vi "LINAKParseStatus.vi"(8 "Error In":errorcluster, 10 "Registers":u16[](array[numeric])) -> (0 "Error Out":errorcluster, 3 "StatusCluster":T1, 4 "GoodToGo":bool)   [LabVIEW 2018]
uses:
  LINAKStatusCluster.ctl
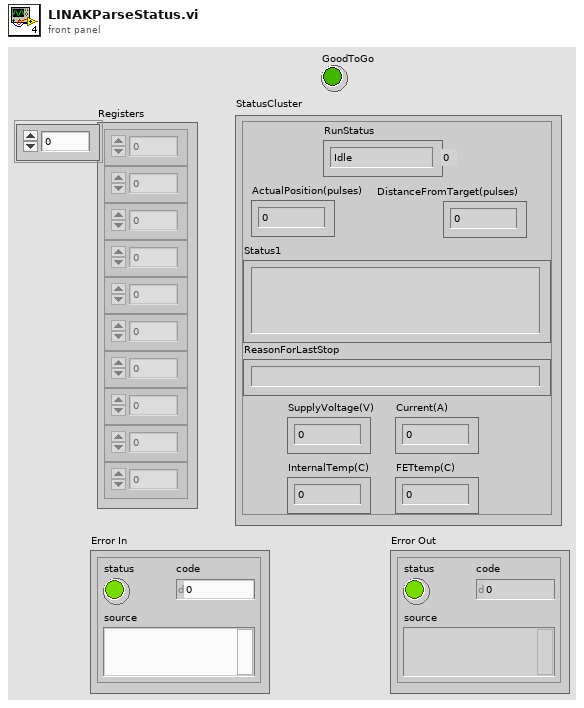
[diagram p1: front panel]
types:
  T1 = typedef "LINAKStatusCluster.ctl" = cluster{"RunStatus":enum16{"Idle", "RunningOut", "RunningIn", "WaitingToRun", "InitOut", "InitIn"}, "ActualPosition(pulses)":u16, "DistanceFromTarget(pulses)":u16, "Status1":string, "ReasonForLastStop":string, "SupplyVoltage(V)":dbl, "Current(A)":dbl, "InternalTemp(C)":i16, "FETtemp(C)":i16}
  T2 = enum16{"Idle", "RunningOut", "RunningIn", "WaitingToRun", "InitOut", "InitIn"}
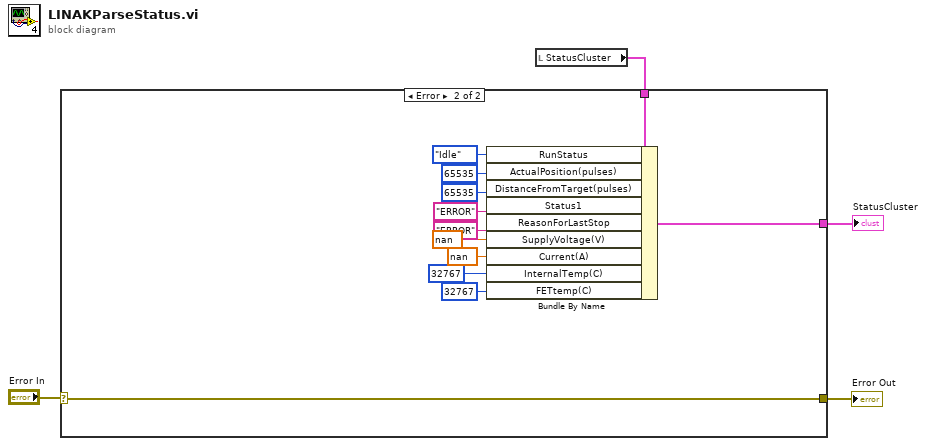
[diagram p0: block diagram]
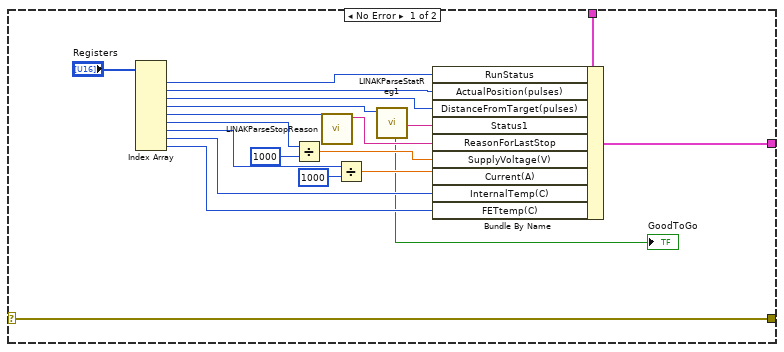
[diagram p2: hidden frame]
diagram:
  n1 = local read "StatusCluster"() -> (w4:T1)
  n2 = case shown="Error" "Error In" {
    selector: "Error In" -> [w5 w25]
    tunnel: w4 -> [w7 w27]
    tunnel: [w6 w26] -> w3
    tunnel: [w5 w25] -> w1
    frame No Error {
      n3 = Index Array(array="Registers") -> (element #1=w22:u16, element #2=w23:u16, element #3=w24:u16, element #4=w20:u16, element #5=w19:u16, element #6=w16:u16, element #7=w12:u16, element #8=w10:u16, element #9=w9:u16)  [unwired: 9 in]
      n4 = Divide(x=w16, y=u16 1000 ("x")) -> (x/y=w15:dbl)
      n5 = call "LINAKParseStopReason.vi"("Numeric Control"=w19) -> ("ReasonForLastStop"=w17:string)  [unwired: 10 in]
      n6 = Divide(x=w12, y=u16 1000 ("x")) -> (x/y=w13:dbl)
      n7 = call "LINAKParseStatReg1.vi"("StatusRegister1"=w20) -> ("StatusString"=w18:string, "GoodToGo"=→"GoodToGo":bool)  [unwired: 6 in, 3 out]
      n8 = Bundle By Name(cluster=w7, "RunStatus"=w22, "ActualPosition(pulses)"=w23, "DistanceFromTarget(pulses)"=w24, "Status1"=w18, "ReasonForLastStop"=w17, "SupplyVoltage(V)"=w15, "Current(A)"=w13, "InternalTemp(C)"=w10, "FETtemp(C)"=w9) -> (w6:T1)
    }
    frame Error {
      n9 = Bundle By Name(cluster=w27, "RunStatus"=T2."Idle", "ActualPosition(pulses)"=u16 65535, "DistanceFromTarget(pulses)"=u16 65535, "Status1"="ERROR", "ReasonForLastStop"="ERROR", "SupplyVoltage(V)"=nan, "Current(A)"=nan, "InternalTemp(C)"=i16 32767, "FETtemp(C)"=i16 32767) -> (w26:T1)
    }
  }
  "Error Out" <- w1
  "StatusCluster" <- w3
